vi "test Scheduled Loopback.vi"(8 "error in":errorcluster, 11 "TestCase in":refnum<class "Single Board 1Ch Loopback.lvclass">) -> (0 "error out":errorcluster, 3 "TestCase out":refnum<class "Single Board 1Ch Loopback.lvclass">)   [LabVIEW 2020, in "Single Board 1Ch Loopback.lvclass"]
uses:
  Single Board 1Ch Loopback.lvclass
  C:/dev/git/niveristand-custom-device-testing-tools/VeriStandTestCase/VeriStandTestCase.lvclass
  <vilib>/numeric/sub_Random U32.vi
  <vilib>/numeric/Random Number (Range) U64.vi
  <vilib>/addons/_JKI Toolkits/VI Tester/TestCase.llb/TestCase.lvclass
  niveristand-custom-device-testing-tools/VeriStandTestUtilities/VeriStandTestUtilities.lvlib
  C:/Program Files (x86)/National Instruments/LabVIEW 2020/vi.lib/addons/_JKI Toolkits/VI Tester/TestCase.llb/TestCase.lvclass
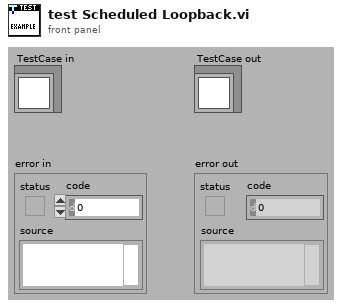
[diagram p1: front panel]
types:
  T1 = typedef "NI_VS Workspace ExecutionAPI.lvlib/WorkspaceAPI.ctl" = refnum<k24>
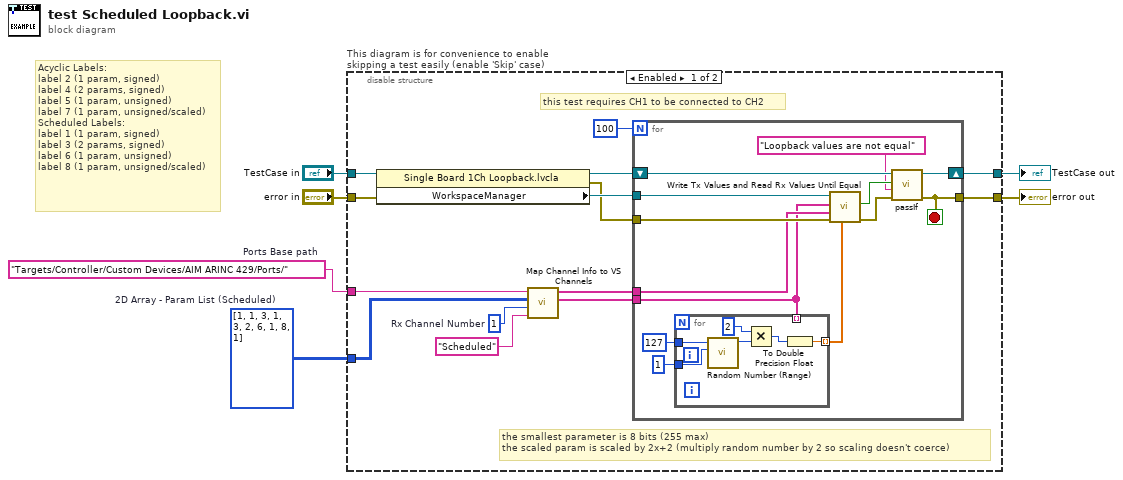
[diagram p0: block diagram]
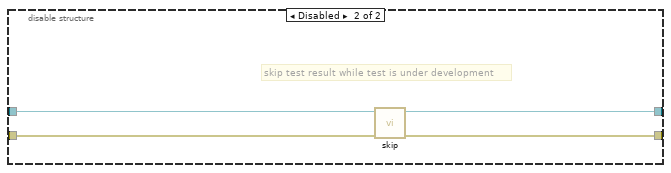
[diagram p2: hidden frame]
diagram:
  w1 = i32[][] [[1, 1], [3, 1], [3, 2], [6, 1], [8, 1]]  # 2D Array - Param List (Scheduled)
  w2 = "Targets/Controller/Custom Devices/AIM ARINC 429/Ports/"  # Ports Base path
  # "Acyclic Labels:\nlabel 2 (1 param, signed)\nlabel 4 (2 params, signed)\nlabel 5 (1 param, unsigned)\nlabel 7 (1 param, unsigned/scaled)\nScheduled Labels:\nlabel 1 (1 param, signed)\nlabel 3 (2 params, signed)\nlabel 6 (1 param, unsigned)\nlabel 8 (1 param, unsigned/scaled)"
  n1 = disable-structure "This diagram is for convenience to enable skipping a test easily (enable 'Skip' case)" shown="Enabled" {
    disable-tunnel: "TestCase in" -> [w14 w43]
    disable-tunnel: [w12 w41] -> w3
    disable-tunnel: [w11 w42] -> w5
    disable-tunnel: "error in" -> [w13 w40]
    disable-tunnel: w2 -> [w15 _]
    disable-tunnel: w1 -> [w8 _]
    frame Enabled {
      w9 = 1  # Rx Channel Number
      # "this test requires CH1 to be connected to CH2"
      # "the smallest parameter is 8 bits (255 max)\nthe scaled param is scaled by 2x+2 (multiply random number by 2 so scaling doesn't coerce)"
      n2 = property class="Single Board 1Ch Loopback.lvcla"(reference=w14, error in=w13) -> (reference out=w17:refnum<class "Single Board 1Ch Loopback.lvclass">, error out=w18:errorcluster, "WorkspaceManager"=w19:T1)
      n3 = call "Map Channel Info to VS Channels.vi"("Transfer Type"="Scheduled", "Rx Channel Number"=w9, "2D Array - Label/Param List"=w8, "VS Channel Base Port"=w15) -> ("Tx Channels Array"=w7:string[], "Rx Channels Array"=w20:string[])  [unwired: 4 in, 2 out]
      n4 = for {
        N: 100 -> [_]
        tunnel: w20 -> [w22]
        tunnel: w19 -> [w33]
        tunnel: w18 -> [w32]
        tunnel: w7 -> [w21]
        shift-right: [w29] -> w12
        shift-left: w17 -> [w30]
        tunnel: [w28] -> w11
        stop <- w28 stop-if-true
        n5 = for {
          tunnel: [w38] -> w23 mode=indexing
          tunnel: u64 127 ("upper bound (100)") -> [w37]
          tunnel: u64 1 ("upper bound (100)") -> [w36]
          tunnel: w21 -> [_] mode=indexing
          n6 = call-poly <vilib>:"Random Number (Range).vi"("lower bound (0)"=w36, "upper bound (100)"=w37) -> ("number"=w39:u64)  [unwired: 9 in]
          n7 = Multiply(x=u64 2, y=w39) -> (x*y=w35:u64)
          n8 = To Double Precision Float(number=w35) -> (double precision float=w38:dbl)
        }
        n9 = call "Write Tx Values and Read Rx Values Until Equal.vi"("Tx values"=w23, "error in"=w32, "Rx aliases"=w22, "Tx aliases"=w21, "workspace manager in"=w33) -> ("error out"=w31:errorcluster, "values equal"=w27:bool)  [unwired: 4 in, 1 out]
        n10 = call-dynamic "passIf.vi"("error in (no error)"=w31, "message (\"\")"="Loopback values are not equal" ("message (\"\")"), "pass"=w27, "TestCase in"=w30) -> ("error out"=w28:errorcluster, "TestCase out"=w29:refnum<class "Single Board 1Ch Loopback.lvclass">)  [unwired: 6 in]
      }
    }
    frame Disabled {
      # "skip test result while test is under development"
      n11 = call <vilib>:"skip.vi"("error in (no error)"=w40, "TestCase in"=w43) -> ("error out"=w42:errorcluster, "TestCase out"=w41:refnum<class "Single Board 1Ch Loopback.lvclass">)  [unwired: 8 in]
    }
  }
  "error out" <- w5
  "TestCase out" <- w3
